vi "Write Name.vi"(8 "error in (no error)":errorcluster, 10 "Name":string, 11 "Type in":refnum<class "Abs_Type.lvclass">) -> (0 "error out":errorcluster, 3 "Type out":refnum<class "Abs_Type.lvclass">)   [LabVIEW 2021, in "Abs_Type.lvclass"]
uses:
  Abs_Type.lvclass
  Abs_Type.lvclass/Abs_Type.ctl
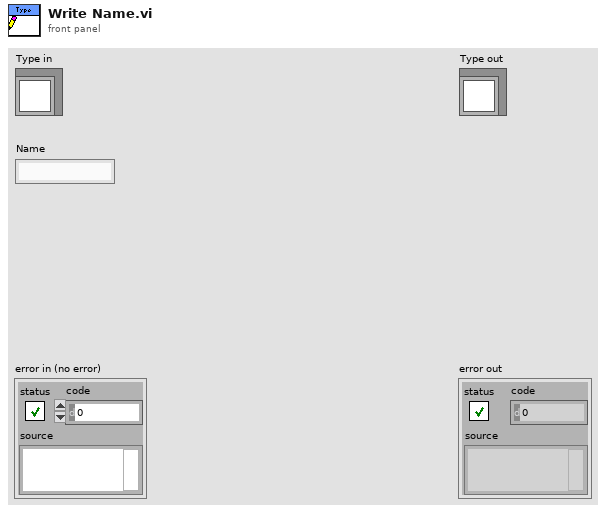
[diagram p1: front panel]
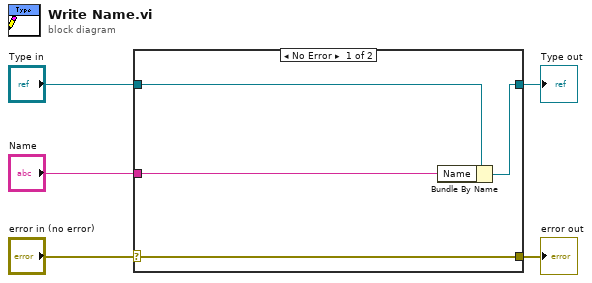
[diagram p0: block diagram]
diagram:
  n1 = case shown="No Error" "error in (no error)" {
    selector: "error in (no error)" -> [w9 w10]
    tunnel: [w9 w10] -> w4
    tunnel: [w7 w11] -> w2
    tunnel: "Type in" -> [w8 w11]
    tunnel: "Name" -> [w6 _]
    frame No Error {
      n2 = Bundle By Name(cluster=w8, "Name"=w6) -> (w7:refnum<class "Abs_Type.lvclass">)
    }
    frame Error {
    }
  }
  "error out" <- w4
  "Type out" <- w2
